vi "DSF.UDP.Transfer.Get IP Address.vi"(8 "error in (no error)":errorcluster, 11 "UDP Transfer in":refnum<class "DSF.UDP.Configuration.Transfer.lvclass">) -> (0 "error out":errorcluster, 2 "IP Address":string="localhost", 3 "UDP Transfer out":refnum<class "DSF.UDP.Configuration.Transfer.lvclass">)   [LabVIEW 2016, in "DSF.UDP.Configuration.Transfer.lvclass"]
uses:
  DSF.UDP.Configuration.Transfer.lvclass
  DSF.UDP.Configuration.Transfer.lvclass/DSF.UDP.Configuration.Transfer.ctl
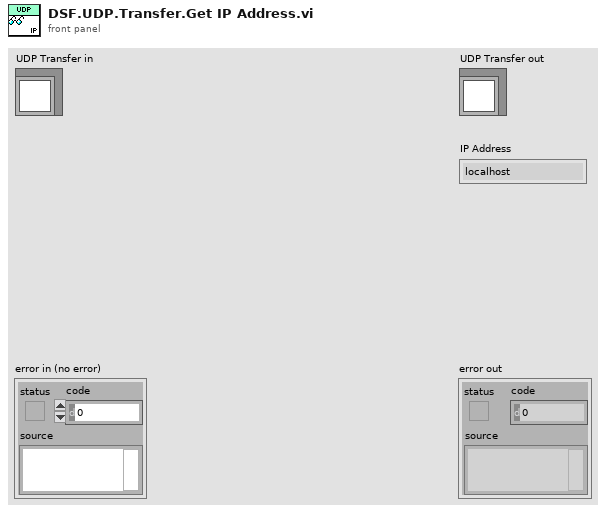
[diagram p1: front panel]
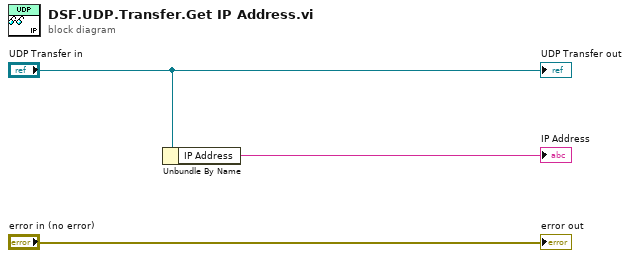
[diagram p0: block diagram]
diagram:
  n1 = Unbundle By Name("UDP Transfer in") -> ("IP Address"=→"IP Address":string)
  "error out" <- "error in (no error)"
  "UDP Transfer out" <- "UDP Transfer in"
